vi "fgv_Reference_Globals.vi"(8 "error in (no error)":errorcluster, 10 "Reference Data":T1={"Refrence data path"=path "", "Reference Rectangle"=[], "AOL Z"=0.0, "No of pixels in a miniscan "=[], "Threshold"=[], "No of miniscans"=[], "Full Frame Size"=0, "Reference Image"=refnum, "dwelltime"=0.1, "Zoom"=1.0, "Field of View"=0.0, "Z Step"=1, "Z pixels"=1, "Z Lines"=1, "Z Ignore"=1, "Laser"=1}, 11 "Function":enum16{"Intialize", "Write", "Read", "Clear"}(ring)) -> (0 "error out":errorcluster, 2 "Reference Data":T1={"Refrence data path"=path "", "Reference Rectangle"=[], "AOL Z"=0.0, "No of pixels in a miniscan "=[], "Threshold"=[], "No of miniscans"=[], "Full Frame Size"=0, "Reference Image"=refnum, "dwelltime"=0.1, "Zoom"=1.0, "Field of View"=0.0, "Z Step"=1, "Z pixels"=1, "Z Lines"=1, "Z Ignore"=1, "Laser"=1})   [LabVIEW 2020]
uses:
  Typedefs/Reference_Globals.ctl
  <vilib>/vision/Image Controls.llb/IMAQ Image.ctl
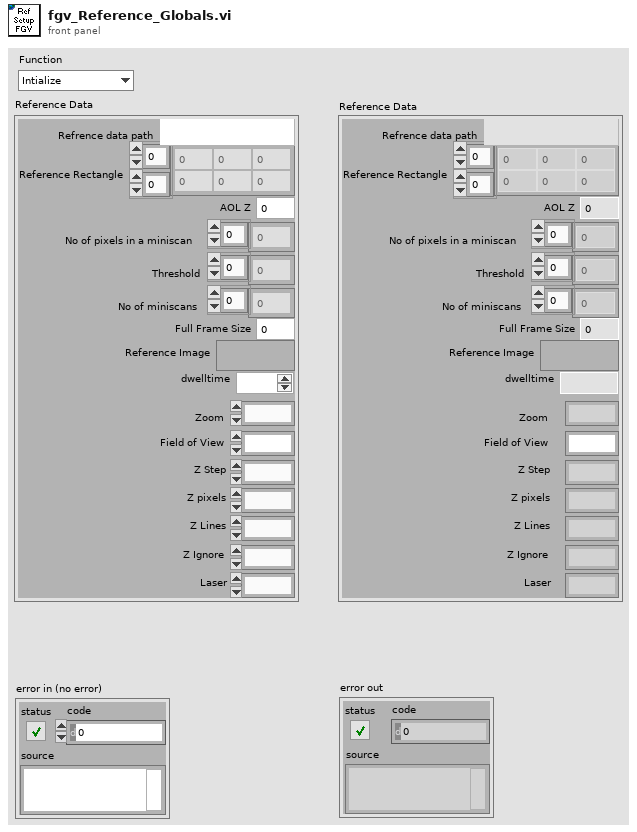
[diagram p1: front panel]
types:
  T1 = typedef "Reference_Globals.ctl" = cluster{"Refrence data path":path, "Reference Rectangle":i16[][], "AOL Z":dbl, "No of pixels in a miniscan ":i32[], "Threshold":i16[], "No of miniscans":i32[], "Full Frame Size":u16, "Reference Image":T2, "dwelltime":dbl, "Zoom":dbl, "Field of View":dbl, "Z Step":i8, "Z pixels":i32, "Z Lines":u8, "Z Ignore":u8, "Laser":u8}
  T2 = typedef "IMAQ Image.ctl" = refnum<image>
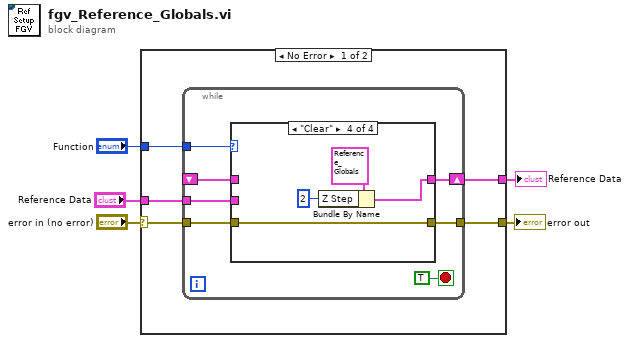
[diagram p0: block diagram]
diagram:
  n1 = case shown="No Error" "error in (no error)" {
    selector: "error in (no error)" -> [w7 w29]
    tunnel: [w8 w29] -> w4
    tunnel: "Function" -> [w10 _]
    tunnel: "Reference Data" -> [w9 w28]
    tunnel: [w6 w28] -> w1
    frame No Error {
      n2 = while {
        tunnel: w10 -> [w16]
        tunnel: w9 -> [w15]
        shift-right: [w14] -> w6
        shift-left: _ -> [w13]
        tunnel: [w11] -> w8
        tunnel: w7 -> [w12]
        stop <- TRUE stop-if-true
        n3 = case shown="\"Clear\"" w16 {
          tunnel: [w19 w21 w23 w25] -> w14
          tunnel: w15 -> [_ w21 _ _]
          tunnel: w13 -> [w19 _ w23 _]
          tunnel: [w18 w20 w22 w27] -> w11
          tunnel: w12 -> [w18 w20 w22 w27]
          frame "Intialize", Default {
          }
          frame "Write" {
          }
          frame "Read" {
          }
          frame "Clear" {
            n4 = Bundle By Name(cluster=T1 {"Refrence data path"=path "", "Reference Rectangle"=[], "AOL Z"=0.0, "No of pixels in a miniscan "=[], "Threshold"=[], "No of miniscans"=[], "Full Frame Size"=0, "Reference Image"=refnum, "dwelltime"=0.0, "Zoom"=0.0, "Field of View"=0.0, "Z Step"=1, "Z pixels"=1, "Z Lines"=1, "Z Ignore"=1, "Laser"=1} ("Reference Data"), "Z Step"=i8 2) -> (w25:T1)
          }
        }
      }
    }
    frame Error {
    }
  }
  "error out" <- w4
  "Reference Data" <- w1
